vi "extScanGlobalVars.vi"() -> ()   [LabVIEW 2014]
panel:
  in  "scanDevTimeout(10ns)":i32
  out "scanDevSet":bool
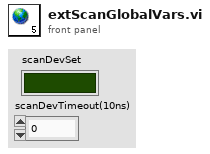
[diagram p1: front panel]
diagram:
